vi "PMU_DATA_PACK.vi"(0 "DATA FRAME":string, 2 "DATA_IN":T2, 3 "PMUs_NUM":u16) -> (6 "PMU DATA Packet":string[](array[string]), 9 "DATA_DTLD":T1)   [LabVIEW 2013]
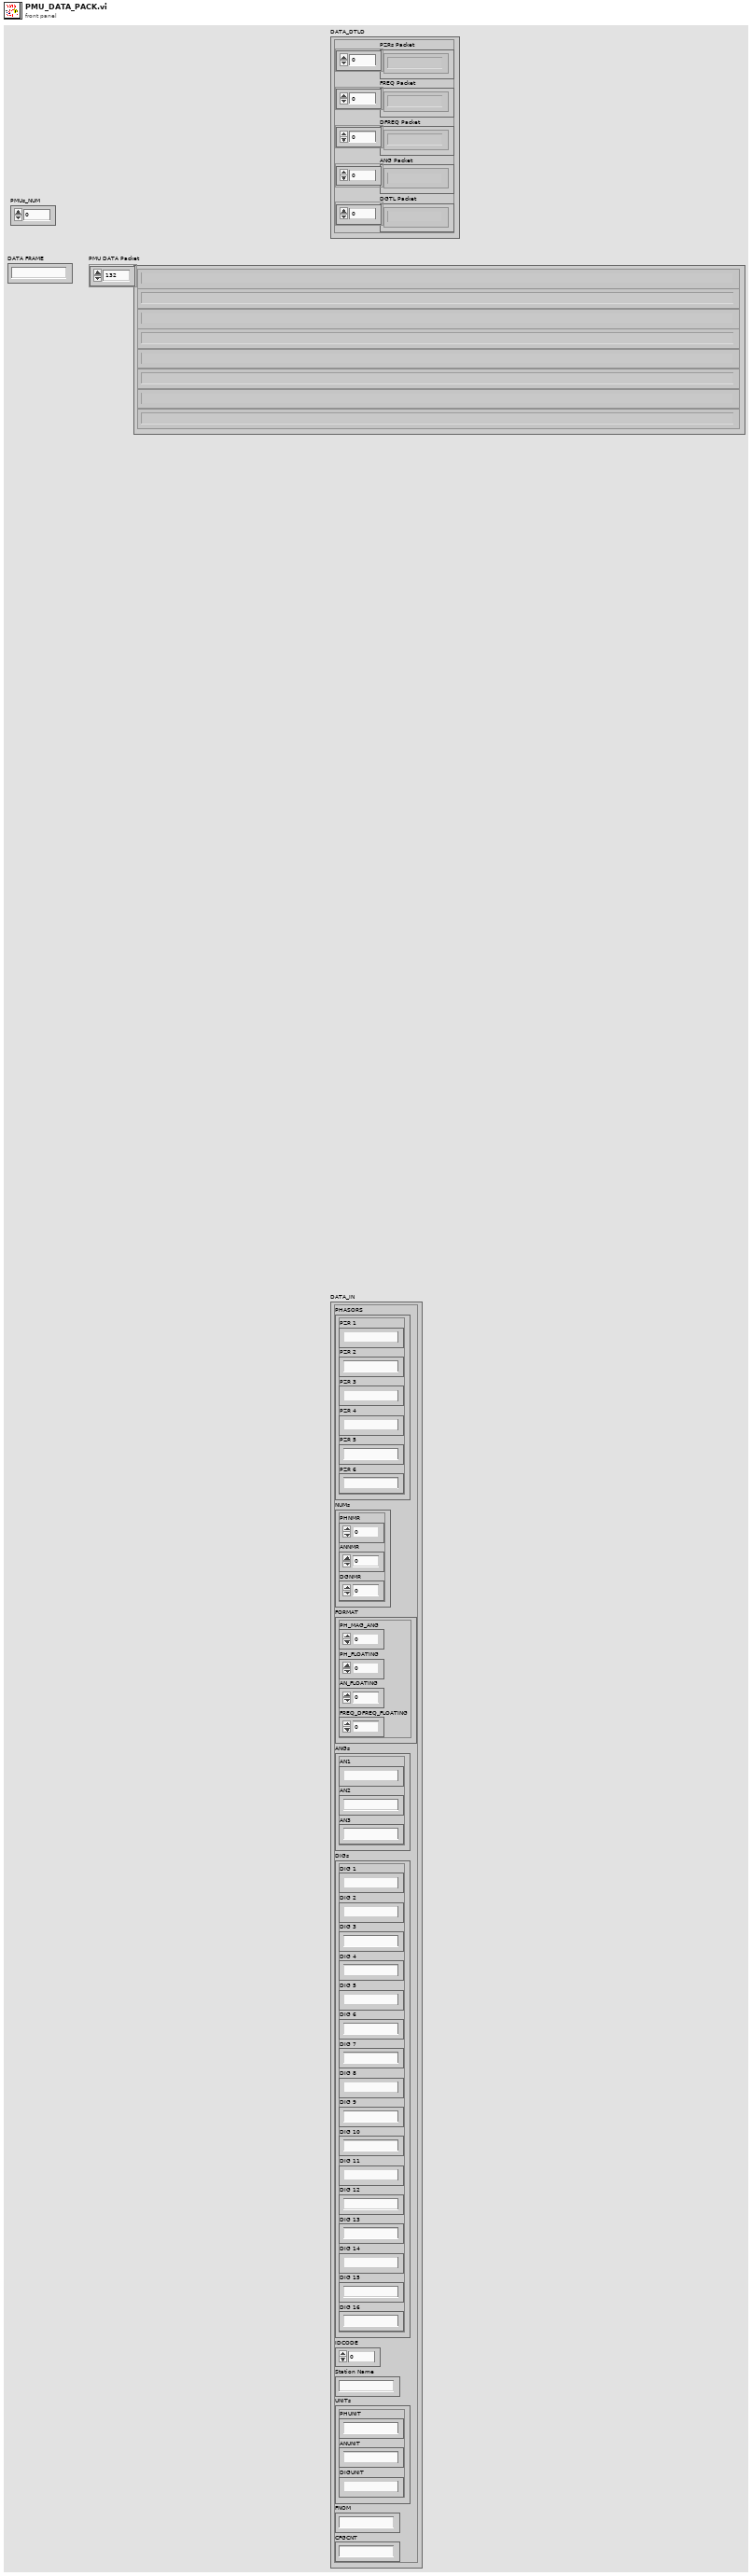
[diagram p1: front panel]
types:
  T1 = cluster{"PZRs Packet":string[], "FREQ Packet":string[], "DFREQ Packet":string[], "ANG Packet":string[], "DGTL Packet":string[]}
  T2 = cluster{"PHASORS":cluster{"PZR 1":string, "PZR 2":string, "PZR 3":string, "PZR 4":string, "PZR 5":string, "PZR 6":string}, "NUMs":cluster{"PHNMR":u8, "ANNMR":u8, "DGNMR":u8}, "FORMAT":cluster{"PH_MAG_ANG":u16, "PH_FLOATING":u16, "AN_FLOATING":u16, "FREQ_DFREQ_FLOATING":u16}, "ANGs":cluster{"AN1":string, "AN2":string, "AN3":string}, "DIGs":cluster{"DIG 1":string, "DIG 2":string, "DIG 3":string, "DIG 4":string, "DIG 5":string, "DIG 6":string, "DIG 7":string, "DIG 8":string, "DIG 9":string, "DIG 10":string, "DIG 11":string, "DIG 12":string, "DIG 13":string, "DIG 14":string, "DIG 15":string, "DIG 16":string}, "IDCODE":u16, "Station Name":string, "UNITs":cluster{"PHUNIT":string, "ANUNIT":string, "DIGUNIT":string}, "FNOM":string, "CFGCNT":string}
  T3 = cluster{"PH_MAG_ANG":u16, "PH_FLOATING":u16, "AN_FLOATING":u16, "FREQ_DFREQ_FLOATING":u16}
  T4 = cluster{"PHNUMR":u16, "ANNUMR":u16, "DGNUMR":u16}
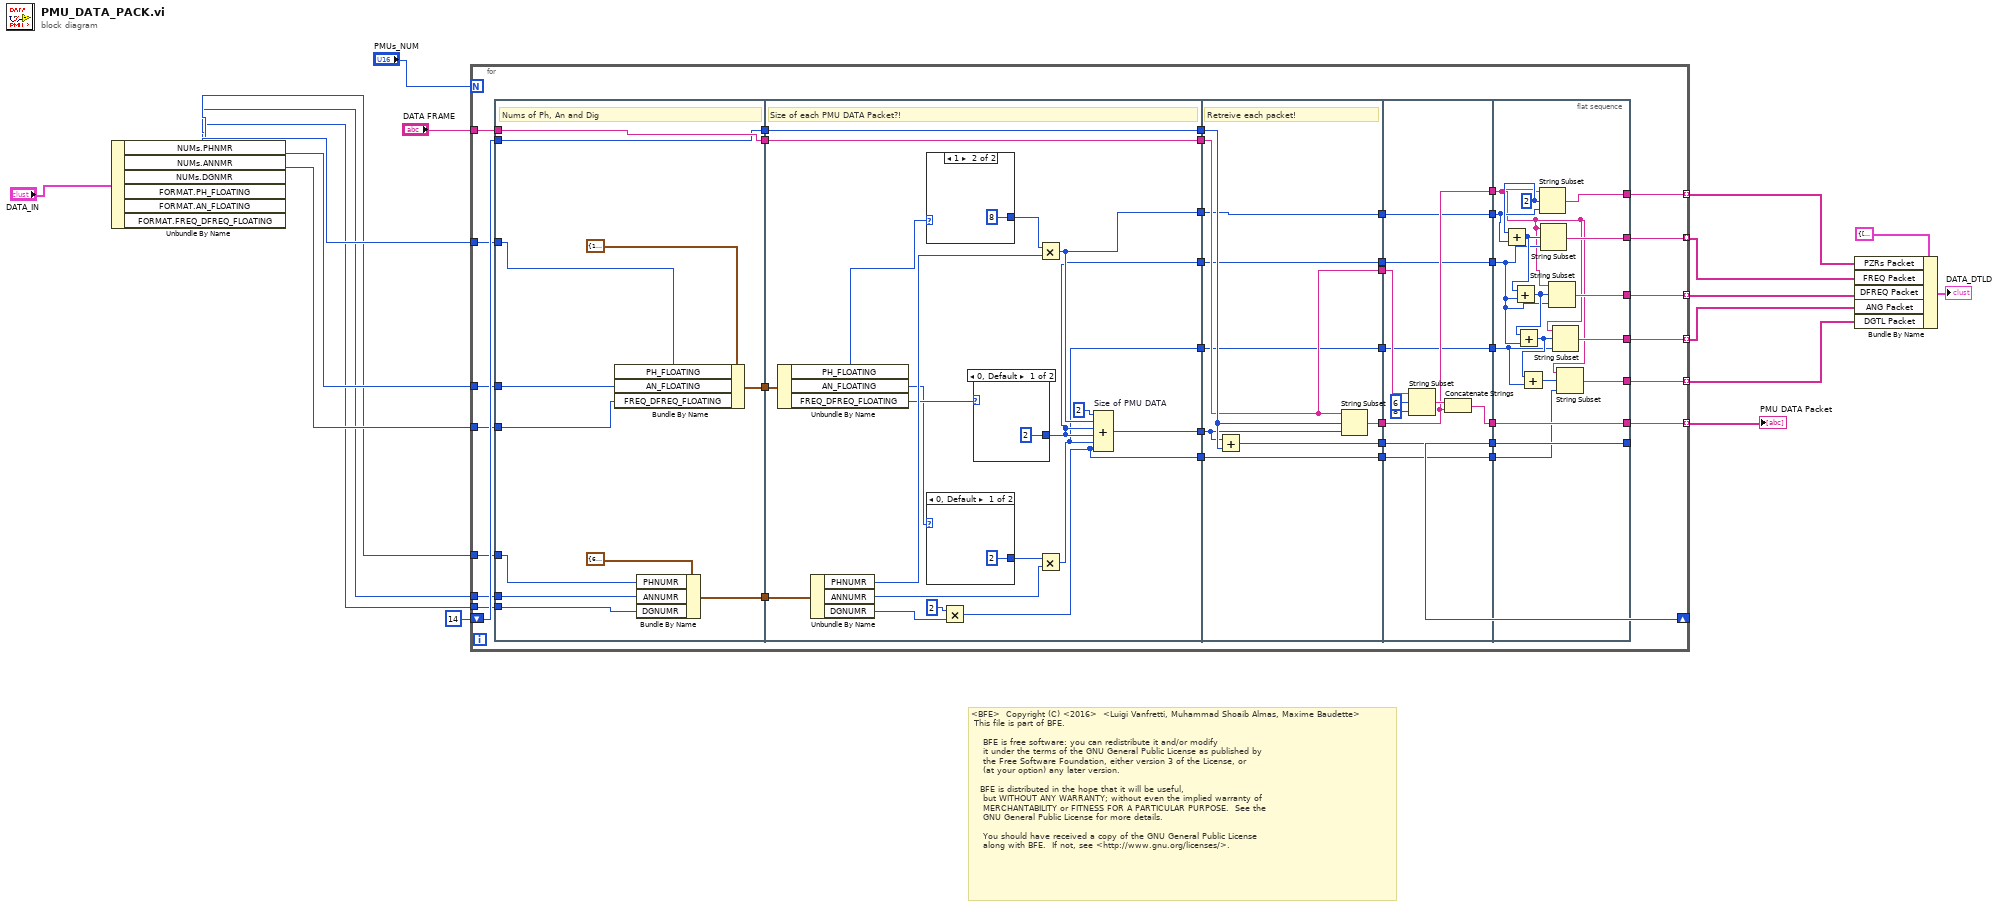
[diagram p0: block diagram]
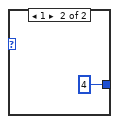
[diagram p2: hidden frame]
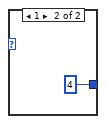
[diagram p3: hidden frame]
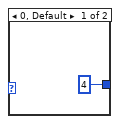
[diagram p4: hidden frame]
diagram:
  # "<BFE>  Copyright (C) <2016>  <Luigi Vanfretti, Muhammad Shoaib Almas, Maxime Baudette>\n This file is part of BFE.\n\n    BFE is free software: you can redistribute it and/or modify\n    it under the terms of the GNU General Public License as published by\n    the Free Software Foundation, either version 3 of the License, or\n    (at your option) any later version.\n\n   BFE is distributed in the hope that it will be useful,\n    but WITHOUT ANY WARRANTY; without even the implied warranty of\n    MERCHANTABILITY or FITNESS FOR A PARTICULAR PURPOSE.  See the\n    GNU General Public License for more details.\n\n    You should have received a copy of the GNU General Public License\n    along with BFE.  If not, see <http://www.gnu.org/licenses/>."
  n1 = Unbundle By Name("DATA_IN") -> ("NUMs.PHNMR"=w11:u8, "NUMs.ANNMR"=w10:u8, "NUMs.DGNMR"=w9:u8, "FORMAT.PH_FLOATING"=w14:u16, "FORMAT.AN_FLOATING"=w13:u16, "FORMAT.FREQ_DFREQ_FLOATING"=w12:u16)
  n2 = for {
    N: "PMUs_NUM" -> [_]
    tunnel: "DATA FRAME" -> [w58]
    shift-right: [w50] -> _
    shift-left: 14 -> [w51]
    tunnel: [w49] -> w17 mode=indexing
    tunnel: w11 -> [w48]
    tunnel: w10 -> [w47]
    tunnel: w9 -> [w46]
    tunnel: w14 -> [w45]
    tunnel: w13 -> [w43]
    tunnel: w12 -> [w42]
    tunnel: [w35] -> w7 mode=indexing
    tunnel: [w31] -> w6 mode=indexing
    tunnel: [w27] -> w5 mode=indexing
    tunnel: [w23] -> w4 mode=indexing
    tunnel: [w22] -> w3 mode=indexing
    n3 = flat-sequence {
      tunnel: w58 -> [w68]
      tunnel: [w69] -> w57
      tunnel: [w68] -> w55
      tunnel: [w67] -> w52
      tunnel: w51 -> [w67]
      tunnel: w48 -> [w66]
      tunnel: w47 -> [w65]
      tunnel: w46 -> [w64]
      tunnel: w45 -> [w61]
      tunnel: [w62] -> w44
      tunnel: w43 -> [w60]
      tunnel: w42 -> [w59]
      tunnel: w57 -> [w89]
      tunnel: [w88] -> w56
      tunnel: w55 -> [w88]
      tunnel: [w86] -> w54
      tunnel: [w87] -> w53
      tunnel: w52 -> [w87]
      tunnel: w44 -> [w82]
      tunnel: [w74] -> w32
      tunnel: [w73] -> w30
      tunnel: [w72] -> w26
      tunnel: [w71] -> w21
      tunnel: w56 -> [w100]
      tunnel: w54 -> [w101]
      tunnel: w53 -> [w103]
      tunnel: [w102] -> w41
      tunnel: [w104] -> w40
      tunnel: [w100] -> w39
      tunnel: [w99] -> w33
      tunnel: w32 -> [w99]
      tunnel: w30 -> [w98]
      tunnel: [w98] -> w29
      tunnel: w26 -> [w97]
      tunnel: [w97] -> w25
      tunnel: w21 -> [w96]
      tunnel: [w96] -> w20
      tunnel: w41 -> [w115]
      tunnel: w40 -> [w109]
      tunnel: w39 -> [w114]
      tunnel: [w115] -> w38
      tunnel: [w112] -> w37
      tunnel: [w109] -> w36
      tunnel: [w108] -> w34
      tunnel: w33 -> [w108]
      tunnel: w29 -> [w107]
      tunnel: [w107] -> w28
      tunnel: w25 -> [w106]
      tunnel: [w106] -> w24
      tunnel: w20 -> [w105]
      tunnel: [w105] -> w19
      tunnel: [w131] -> w49
      tunnel: [w132] -> w50
      tunnel: w38 -> [w132]
      tunnel: w37 -> [w131]
      tunnel: w36 -> [w116]
      tunnel: [w130] -> w35
      tunnel: w34 -> [w127]
      tunnel: [w129] -> w31
      tunnel: w28 -> [w123]
      tunnel: [w125] -> w27
      tunnel: w24 -> [w119]
      tunnel: [w122] -> w23
      tunnel: [w118] -> w22
      tunnel: w19 -> [w117]
      frame #0 {
        # "Nums of Ph, An and Dig"
        n4 = Bundle By Name(cluster=T3 {"PH_MAG_ANG"=1, "PH_FLOATING"=2, "AN_FLOATING"=4, "FREQ_DFREQ_FLOATING"=8}, "PH_FLOATING"=w61, "AN_FLOATING"=w60, "FREQ_DFREQ_FLOATING"=w59) -> (w62:T3)
        n5 = Bundle By Name(cluster=T4 {"PHNUMR"=6, "ANNUMR"=3, "DGNUMR"=1}, "PHNUMR"=w66, "ANNUMR"=w65, "DGNUMR"=w64) -> (w69:T4)
      }
      frame #1 {
        # "Size of each PMU DATA Packet?!"
        n6 = Unbundle By Name(w82) -> ("PH_FLOATING"=w81:u16, "AN_FLOATING"=w79:u16, "FREQ_DFREQ_FLOATING"=w80:u16)
        n7 = Unbundle By Name(w89) -> ("PHNUMR"=w83:u16, "ANNUMR"=w77:u16, "DGNUMR"=w75:u16)
        n8 = case shown="1" w81 {
          tunnel: [u8 4 ("value") u8 8 ("value")] -> w84
          frame 0, Default {
          }
          frame 1 {
          }
        }
        n9 = case shown="0, Default" w79 {
          tunnel: [u8 2 ("value") u8 4 ("value")] -> w78
          frame 0, Default {
          }
          frame 1 {
          }
        }
        n10 = Multiply(x=u8 2 ("value"), y=w75) -> (x*y=w71:u16)
        n11 = case shown="0, Default" w80 {
          tunnel: [u8 2 ("value") u8 4 ("value")] -> w73
          frame 0, Default {
          }
          frame 1 {
          }
        }
        n12 = Multiply(x=w84, y=w83) -> (x*y=w74:u16)
        n13 = Multiply(x=w78, y=w77) -> (x*y=w72:u16)
        n14 = Compound Arithmetic op=ADD "Size of PMU DATA"(u8 2 ("value"), w74, w73, w73, w72, w71) -> (w86:u16)
      }
      frame #2 {
        # "Retreive each packet!"
        n15 = Add(x=w101, y=w103) -> (x+y=w102:i32)
        n16 = String Subset(string=w100, offset (0)=w103, length (rest)=w101) -> (substring=w104:string)
      }
      frame #3 {
        n17 = String Subset(string=w114, offset (0)=6, length (rest)=8 ("length (rest)")) -> (substring=w113:string)
        n18 = Concatenate Strings(w113, w109) -> (w112:string)
      }
      frame #4 {
        w128 = 2 ("offset (0)")
        n19 = Add(x=w128, y=w127) -> (x+y=w126:i32)
        n20 = Add(x=w126, y=w123) -> (x+y=w124:i32)
        n21 = Add(x=w124, y=w123) -> (x+y=w120:i32)
        n22 = Add(x=w120, y=w119) -> (x+y=w121:i32)
        n23 = String Subset(string=w116, offset (0)=w128, length (rest)=w127) -> (substring=w130:string)
        n24 = String Subset(string=w116, offset (0)=w126, length (rest)=w123) -> (substring=w129:string)
        n25 = String Subset(string=w116, offset (0)=w124, length (rest)=w123) -> (substring=w125:string)
        n26 = String Subset(string=w116, offset (0)=w120, length (rest)=w119) -> (substring=w122:string)
        n27 = String Subset(string=w116, offset (0)=w121, length (rest)=w117) -> (substring=w118:string)
      }
    }
  }
  "PMU DATA Packet" <- w17
  n28 = Bundle By Name(cluster=T1 {"PZRs Packet"=[], "FREQ Packet"=[], "DFREQ Packet"=[], "ANG Packet"=[], "DGTL Packet"=[]}, "PZRs Packet"=w7, "FREQ Packet"=w6, "DFREQ Packet"=w5, "ANG Packet"=w4, "DGTL Packet"=w3) -> (→"DATA_DTLD":T1)
